vi "OOBSeqReport.vi"(8 "error in (no error)":errorcluster, 11 "Array":string[][](array[string])) -> (0 "error out":errorcluster)   [LabVIEW 2014]
uses:
  typedefs/ePathsAction.ctl
  Excel(ActiveX)/enumOpenOrCreate.ctl
  Excel(ActiveX)/Excel(ActiveX).lvlib
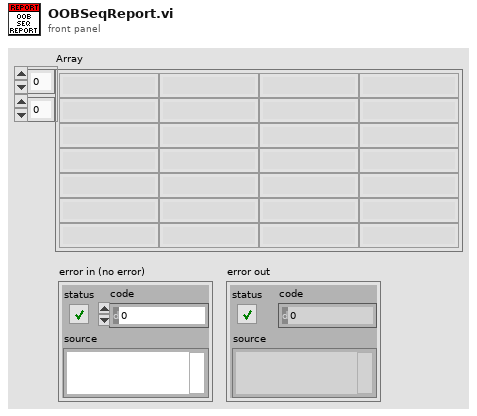
[diagram p1: front panel]
types:
  T1 = typedef "Excel(ActiveX).lvlib/enumOpenOrCreate.ctl" = enum16{"open", "open or create", "create from template"}
  T2 = typedef "ePathsAction.ctl" = enum16{"Set", "Get", "Load", "Save", "Default", "Exit"}
  T3 = typedef "Paths.ctl" = cluster{"BasePath":path, "CutPath":path, "LastCutPath":path, "CCSPath":path, "LastCCSPath":path, "ResultsPath":path}
  T4 = typedef "Excel(ActiveX).lvlib/ExcelActiveX.ctl" = cluster{"Excel._Application":refnum<k7>, "Application open at start":bool, "Excel._Worksheet":refnum<k7>, "Workbook open at start":bool, "Excel._Workbook":refnum<k7>, "Workbook Path":path, "Worksheet Name":string, "Row":u32, "Col":u32, "Cell":string, "Workbook Name":string}
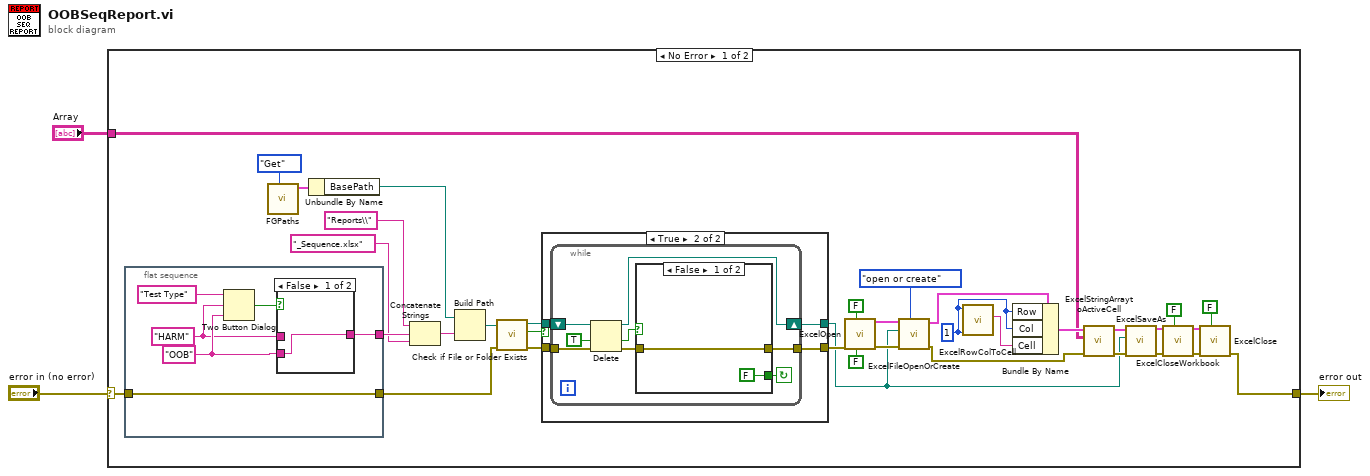
[diagram p0: block diagram]
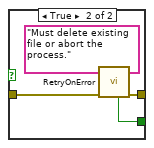
[diagram p3: hidden frame]
diagram:
  n1 = case shown="No Error" "error in (no error)" {
    selector: "error in (no error)" -> [w36 w67]
    tunnel: [w5 w67] -> w2
    tunnel: "Array" -> [w14 _]
    frame No Error {
      w17 = u32 1 ("col")
      n2 = flat-sequence {
        tunnel: [w60] -> w26
        tunnel: w36 -> [w60]
        tunnel: [w59] -> w35
        frame #0 {
          w62 = "OOB" ("message")
          w61 = "HARM" ("message")
          n3 = Two Button Dialog(message="Test Type", 1:w62, 2:w61) -> (T button?=w63:bool)
          n4 = case shown="False" w63 {
            tunnel: w62 -> [w65 _]
            tunnel: w61 -> [_ w66]
            tunnel: [w65 w66] -> w59
            frame False {
            }
            frame True {
            }
          }
        }
      }
      n5 = call "FGPaths.vi"("ePathsAction"=ePathsAction."Get") -> ("PathsOut"=w37:T3)  [unwired: 9 in, 1 out]
      n6 = Unbundle By Name(w37) -> ("BasePath"=w32:path)
      n7 = Concatenate Strings("Reports\\" ("message"), w35, "_Sequence.xlsx" ("message")) -> (w31:string)
      n8 = Build Path(base path=w32, name or relative path=w31) -> (appended path=w27:path)
      n9 = call <vilib>:"Check if File or Folder Exists.vi"("error in (no error)"=w26, "path"=w27) -> ("error out"=w28:errorcluster, "file or folder exists?"=w30:bool, "dup path"=w29:path)  [unwired: 7 in]
      n10 = case shown="True" w30 {
        tunnel: w29 -> [w39 w44]
        tunnel: w28 -> [w40 w43]
        tunnel: [w40 w41] -> w21
        tunnel: [w39 w42] -> w4
        frame False {
        }
        frame True {
          n11 = while {
            shift-right: [w49] -> w42
            shift-left: w44 -> [w51]
            tunnel: w43 -> [w50]
            tunnel: [w47] -> w41
            stop <- w45 continue-if-true
            n12 = Delete(path (use dialog)=w51, confirm (F)=TRUE, error in=w50) -> (deleted path=w49:path, cancelled=w46:bool, error out=w48:errorcluster)  [unwired: 2 in]
            n13 = case shown="False" w46 {
              tunnel: w48 -> [w54 w56]
              tunnel: [w54 w58] -> w47
              tunnel: [FALSE ("Retry") w57] -> w45
              frame False {
              }
              frame True {
                n14 = call "RetryOnError.vi"("error in (no error)"=w56, "Error Msg"="Must delete existing file or abort the process.") -> ("error out"=w58:errorcluster, "Retry"=w57:bool)  [unwired: 8 in]
              }
            }
          }
        }
      }
      n15 = call "ExcelOpen.vi"("Run Minimized (f)"=FALSE, "Excel visible? (t)"=FALSE, "error in (no error)"=w21) -> ("error out"=w24:errorcluster, "ExcelActiveX"=w25:T4)  [unwired: 7 in]
      n16 = call "ExcelFileOpenOrCreate.vi"("Open or Create"=enumOpenOrCreate."open or create", "error in (no error)"=w24, "Excel file name and path"=w4, "ExcelActiveX in"=w25) -> ("error out"=w16:errorcluster, "ExcelActiveX out"=w19:T4)  [unwired: 6 in]
      n17 = call "ExcelRowColToCell.vi"("col"=w17, "row"=w17) -> ("cell"=w18:string)  [unwired: 9 in]
      n18 = Bundle By Name(cluster=w19, "Row"=w17, "Col"=w17, "Cell"=w18) -> (w15:T4)
      n19 = call "ExcelStringArraytoActiveCell.vi"("error in (no error)"=w16, "Array"=w14, "ExcelActiveX"=w15) -> ("error out"=w7:errorcluster, "ExcelActiveX"=w6:T4)  [unwired: 7 in]
      n20 = call "ExcelSaveAs.vi"("error in (no error)"=w7, "Path"=w4, "ExcelActiveX"=w6) -> ("error out"=w12:errorcluster, "ExcelActiveX"=w10:T4)  [unwired: 7 in]
      n21 = call "ExcelCloseWorkbook.vi"("Save"=FALSE, "error in (no error)"=w12, "ExcelActiveX"=w10) -> ("error out"=w11:errorcluster, "ExcelActiveX"=w9:T4)  [unwired: 7 in]
      n22 = call "ExcelClose.vi"("Leave Open (f)"=FALSE, "error in (no error)"=w11, "ExcelActiveX in"=w9) -> ("error out"=w5:errorcluster)  [unwired: 7 in, 1 out]
    }
    frame Error {
    }
  }
  "error out" <- w2
